vi "청기백기 (1).vi"() -> ()   [LabVIEW 2013]
panel:
  out "틀린횟수":i32
  in  "백기":bool
  in  "청기":bool
  out "청기 백기":string
  in  "게임시작":string
  in  "안내문":string
  out "시간":i32
  out "백기":bool=TRUE
  out "청기":bool=TRUE
  in  "정지":bool
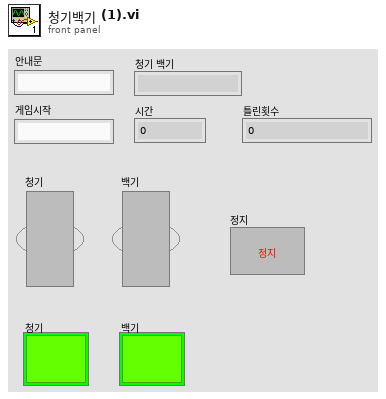
[diagram p1: front panel]
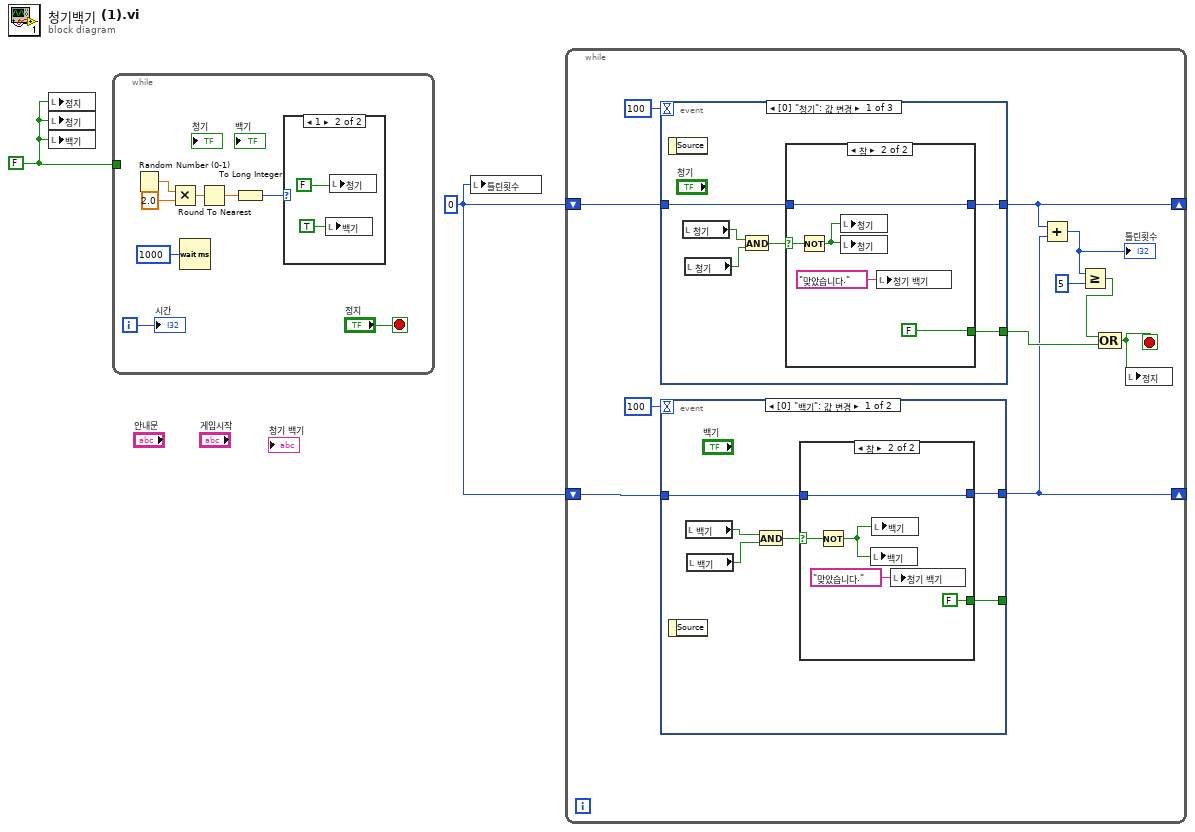
[diagram p0: block diagram]
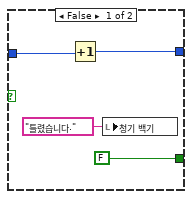
[diagram p2: hidden frame]
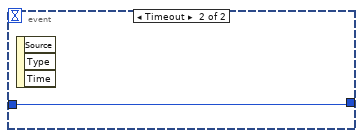
[diagram p3: hidden frame]
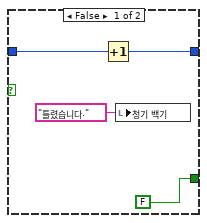
[diagram p4: hidden frame]
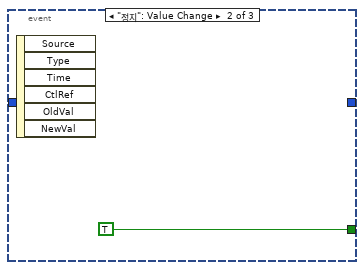
[diagram p5: hidden frame]
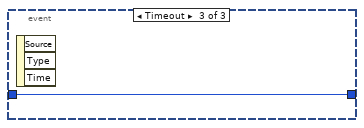
[diagram p6: hidden frame]
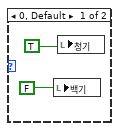
[diagram p7: hidden frame]
diagram:
  w1 = FALSE ("정지")
  w2 = 0
  n1 = local write "정지"(w1) -> ()
  n2 = local write "청기"(w1) -> ()
  n3 = local write "백기"(w1) -> ()
  n4 = while {
    tunnel: w1 -> [_]
    i -> [w3]
    stop <- "정지" stop-if-true
    n5 = Random Number (0-1)() -> (number: 0 to 1=w10:dbl)
    n6 = Multiply(x=w10, y=2.0) -> (x*y=w8:dbl)
    n7 = Wait (ms)(milliseconds to wait=u32 1000 ("대기 시간(ms)")) -> ()  [unwired: 1 out]
    n8 = Round To Nearest(number=w8) -> (nearest integer value=w6:dbl)
    n9 = To Long Integer(number=w6) -> (32bit integer=w5:i32)
    n10 = case shown="1" w5 {
      frame 0, Default {
        n11 = local write "백기"(FALSE) -> ()
        n12 = local write "청기"(TRUE) -> ()
      }
      frame 1 {
        n13 = local write "백기"(TRUE) -> ()
        n14 = local write "청기"(FALSE) -> ()
      }
    }
    "시간" <- w3
  }
  n15 = local write "틀린횟수"(w2) -> ()
  n16 = while {
    shift-right: [w19] -> _
    shift-left: w2 -> [w25]
    shift-right: [w18] -> _
    shift-left: w2 -> [w20]
    stop <- w23 stop-if-true
    n17 = event shown="[0] \"청기\": 값 변경" {
      selector: _ -> [_ _ _]
      dyn-events: _ -> [_ _ _]
      timeout: 100 -> [_ _ _]
      tunnel: [w45 TRUE _] -> w24
      tunnel: w25 -> [w43 _ w58]
      tunnel: [w42 _ w58] -> w19
      event "청기": Value Change {
        n18 = event-data() -> ()  [unwired: 1 in, 1 out]
        n19 = local read "청기"() -> (w44:bool)
        n20 = local read "청기"() -> (w47:bool)
        n21 = And(x=w44, y=w47) -> (x .and. y?=w46:bool)
        n22 = case shown="참" w46 {
          selector: w46 -> [_ w56]
          tunnel: [FALSE FALSE] -> w45
          tunnel: w43 -> [w49 w52]
          tunnel: [w48 w52] -> w42
          frame False {
            n23 = Increment(x=w49) -> (x+1=w48:i32)
            n24 = local write "청기 백기"("틀렸습니다." ("청기 백기")) -> ()
          }
          frame True {
            n25 = Not(x=w56) -> (.not. x?=w55:bool)
            n26 = local write "청기"(w55) -> ()
            n27 = local write "청기"(w55) -> ()
            n28 = local write "청기 백기"("맞았습니다." ("청기 백기")) -> ()
          }
        }
      }
      event "정지": Value Change {
        n29 = event-data() -> ()  [unwired: 1 in, 6 out]
      }
      event Timeout {
        n30 = event-data() -> ()  [unwired: 1 in, 3 out]
      }
    }
    n31 = event shown="[0] \"백기\": 값 변경" {
      selector: _ -> [_ _]
      dyn-events: _ -> [_ _]
      timeout: 100 -> [_ _]
      tunnel: [w30 _] -> _
      tunnel: w20 -> [w27 w41]
      tunnel: [w26 w41] -> w18
      event "백기": Value Change {
        n32 = event-data() -> ()  [unwired: 1 in, 1 out]
        n33 = local read "백기"() -> (w28:bool)
        n34 = local read "백기"() -> (w29:bool)
        n35 = And(x=w28, y=w29) -> (x .and. y?=w31:bool)
        n36 = case shown="참" w31 {
          selector: w31 -> [_ w40]
          tunnel: [FALSE FALSE] -> w30
          tunnel: w27 -> [w33 w36]
          tunnel: [w32 w36] -> w26
          frame False {
            n37 = Increment(x=w33) -> (x+1=w32:i32)
            n38 = local write "청기 백기"("틀렸습니다." ("청기 백기")) -> ()
          }
          frame True {
            n39 = Not(x=w40) -> (.not. x?=w39:bool)
            n40 = local write "백기"(w39) -> ()
            n41 = local write "백기"(w39) -> ()
            n42 = local write "청기 백기"("맞았습니다." ("청기 백기")) -> ()
          }
        }
      }
      event Timeout {
        n43 = event-data() -> ()  [unwired: 1 in, 3 out]
      }
    }
    n44 = Add(x=w19, y=w18) -> (x+y=w17:i32)
    "틀린횟수" <- w17
    n45 = Greater Or Equal?(x=w17, y=5) -> (x >= y?=w21:bool)
    n46 = Compound Arithmetic op=OR(w21, w24) -> (w23:bool)
    n47 = local write "정지"(w23) -> ()
  }
